vi "CANOpen TPDOs.vi"(8 "error in (no error)":errorcluster, 11 "Node Ptr":T1 format="%.0x") -> (0 "error out":errorcluster)   [LabVIEW 2013, in "CANOpen Addon Custom Device.lvlib"]
uses:
  CANOpen Addon Custom Device.lvlib
  <vilib>/NI Veristand/Custom Device API/Custom Device Item Ref.ctl
  <vilib>/NI Veristand/Custom Device API/Custom Device API.lvlib
panel:
  in  "SHDocVw.IWebBrowser2":refnum<k7>(container)
  in  "Header":cluster{"Section Name":string}={"Section Name"="TPDOs"}
  in  "Description":string
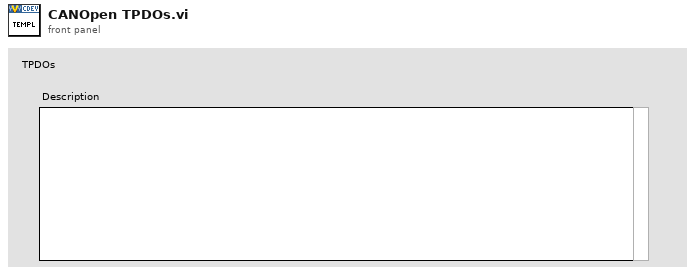
[diagram p1: front panel]
types:
  T1 = typedef "Custom Device API.lvlib/Custom Device Item Ref.ctl" = u64
  T2 = typedef "Custom Device API.lvlib/Custom Device Commands.ctl" = enum16{"Default", "Item renamed", "Shutdown", "Dynamic button pressed"}
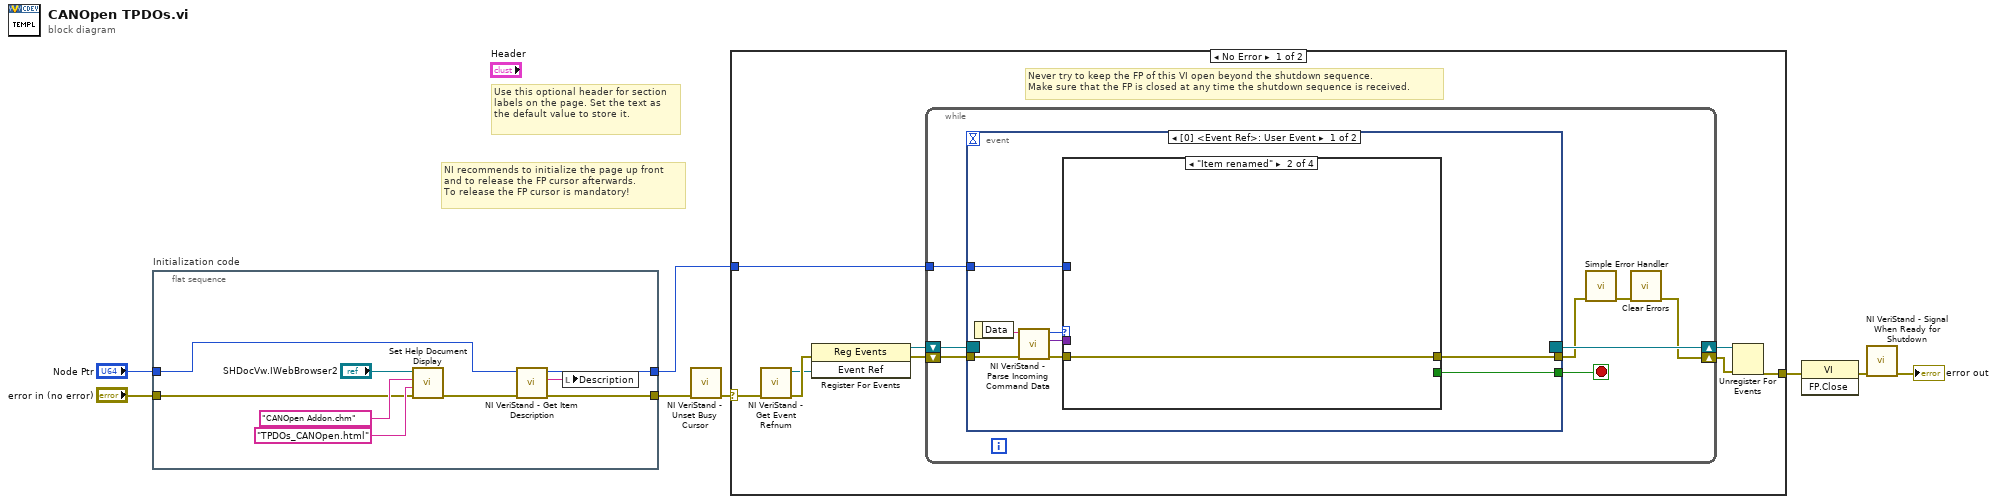
[diagram p0: block diagram]
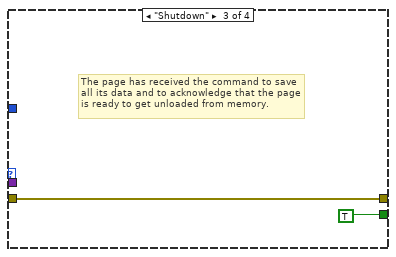
[diagram p3: hidden frame]
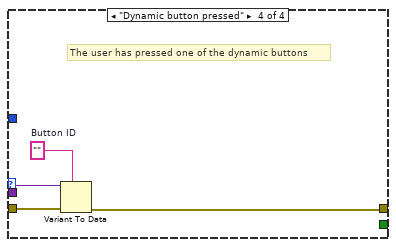
[diagram p4: hidden frame]
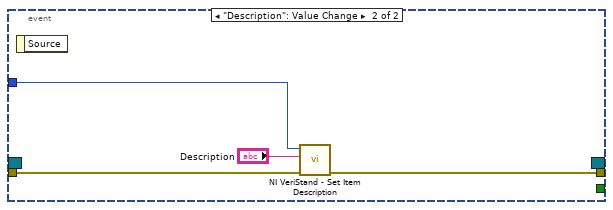
[diagram p5: hidden frame]
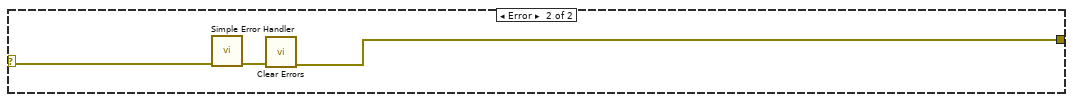
[diagram p6: hidden frame]
diagram:
  # "Use this optional header for section labels on the page. Set the text as the default value to store it."
  # "NI recommends to initialize the page up front\nand to release the FP cursor afterwards.\nTo release the FP cursor is mandatory!"
  n1 = flat-sequence "Initialization code" {
    tunnel: "error in (no error)" -> [w10]
    tunnel: "Node Ptr" -> [w17]
    tunnel: [w15] -> w4
    tunnel: [w14] -> w1
    frame #0 {
      n2 = call "Set Help Document Display.vi"("error in (no error)"=w10, "HTML File"="TPDOs_CANOpen.html", "Main CHM File"="CANOpen Addon.chm", "SHDocVw.IWebBrowser2"="SHDocVw.IWebBrowser2") -> ("error out"=w9:errorcluster)  [unwired: 7 in]
      n3 = call <vilib>:"NI VeriStand - Get Item Description.vi"("error in (no error)"=w9, "Item Ref in"=w17) -> ("error out"=w15:errorcluster, "Description"=w16:string, "Item Ref out"=w14:T1)  [unwired: 7 out]
      n4 = local write "Description"(w16) -> ()
    }
  }
  n5 = call <vilib>:"NI VeriStand - Unset Busy Cursor.vi"("error in (no error)"=w4) -> ("error out"=w3:errorcluster)  [unwired: 10 out]
  n6 = case shown="No Error" w3 {
    selector: w3 -> [w18 w57]
    tunnel: [w23 w55] -> w8
    tunnel: w1 -> [w19 _]
    frame No Error {
      # "Never try to keep the FP of this VI open beyond the shutdown sequence.\nMake sure that the FP is closed at any time the shutdown sequence is received."
      n7 = call <vilib>:"NI VeriStand - Get Event Refnum.vi"("error in (no error)"=w18) -> ("error out"=w26:errorcluster, "Event Ref"=w22:refnum<user-event>)  [unwired: 9 out]
      n8 = register-events(error in=w26, w22) -> (reference out=w20:refnum<event-registration>, error out=w21:errorcluster)  [unwired: 1 in]
      n9 = while {
        tunnel: w19 -> [w30]
        shift-right: [w27] -> w24
        shift-left: w21 -> [w33]
        shift-right: [w34] -> w25
        shift-left: w20 -> [w32]
        stop <- w31 stop-if-true
        n10 = event shown="[0] <Event Ref>: User Event" {
          selector: w32 -> [_ _]
          dyn-events: [_ _] -> w34
          timeout: _ -> [_ _]
          tunnel: w33 -> [w42 w53]
          tunnel: [w38 _] -> w31
          tunnel: [w37 w52] -> w29
          tunnel: w30 -> [w36 w54]
          event User Event {
            n11 = event-data() -> ("Data"=w41:string)  [unwired: 1 out]
            n12 = call <vilib>:"NI VeriStand - Parse Incoming Command Data.vi"("error in (no error)"=w42, "Incoming data"=w41) -> ("error out"=w40:errorcluster, "Outgoing data"=w35:variant, "Action"=w39:T2)  [unwired: 7 out]
            n13 = case shown="\"Item renamed\"" w39 {
              tunnel: w40 -> [w43 w44 w45 w50]
              tunnel: [_ _ TRUE _] -> w38
              tunnel: [w43 w44 w45 w47] -> w37
              tunnel: w36 -> [_ _ _ _]
              tunnel: w35 -> [_ _ _ w49]
              frame "Default", Default {
              }
              frame "Item renamed" {
              }
              frame "Shutdown" {
                # "The page has received the command to save all its data and to acknowledge that the page is ready to get unloaded from memory."
              }
              frame "Dynamic button pressed" {
                w48 = ""  # Button ID
                # "The user has pressed one of the dynamic buttons"
                n14 = Variant To Data(error in=w50, type=w48, Variant=w49) -> (error out=w47:errorcluster)  [unwired: 1 out]
              }
            }
          }
          event "Description": Value Change {
            n15 = event-data() -> ()  [unwired: 2 out]
            n16 = call <vilib>:"NI VeriStand - Set Item Description.vi"("error in (no error)"=w53, "Description"="Description", "Item Ref in"=w54) -> ("error out"=w52:errorcluster)  [unwired: 8 out]
          }
        }
        n17 = call <vilib>:"Simple Error Handler.vi"("error in (no error)"=w29) -> ("error out"=w28:errorcluster)  [unwired: 1 in, 7 out]
        n18 = call <vilib>:"Clear Errors.vi"("error in (no error)"=w28) -> ("error out"=w27:errorcluster)  [unwired: 6 out]
      }
      n19 = Unregister For Events(event registration refnum=w25, error in=w24) -> (error out=w23:errorcluster)
    }
    frame Error {
      n20 = call <vilib>:"Simple Error Handler.vi"("error in (no error)"=w57) -> ("error out"=w56:errorcluster)  [unwired: 1 in, 7 out]
      n21 = call <vilib>:"Clear Errors.vi"("error in (no error)"=w56) -> ("error out"=w55:errorcluster)  [unwired: 6 out]
    }
  }
  n22 = invoke class="VI" method="FP.Close"(error in=w8) -> (error out=w7:errorcluster)  [unwired: 2 in, 2 out]
  n23 = call <vilib>:"NI VeriStand - Signal When Ready for Shutdown.vi"("error in (no error)"=w7) -> ("error out"=→"error out":errorcluster)  [unwired: 10 out]
